vi "String to I8.vi"(8 "Error In":errorcluster, 11 "String":string) -> (0 "Error Out":errorcluster, 2 "I8":i8, 3 "rest of String":string)   [LabVIEW 2011, in "Tinkerforge.lvlib" / "Device.lvclass"]
doc: "This VI converts a binary little-endian I8 string into a numeric I8."
uses:
  Device.lvclass
  IP Connection/IP Connection.lvclass
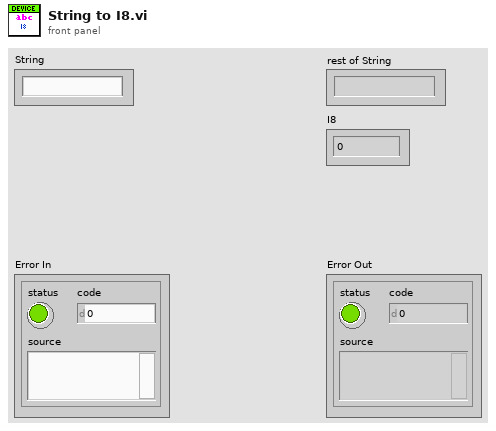
[diagram p1: front panel]
types:
  T1 = enum16{"big-endian, network order", "native, host order", "little-endian"}
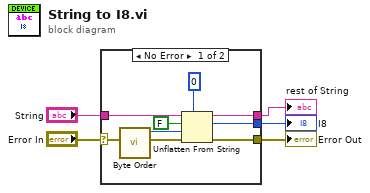
[diagram p0: block diagram]
diagram:
  n1 = case shown="No Error" "Error In" {
    selector: "Error In" -> [w12 w15]
    tunnel: "String" -> [w9 w14]
    tunnel: [w8 w15] -> w3
    tunnel: [w7 _] -> w2
    tunnel: [w6 w14] -> w1
    frame No Error {
      n2 = call "Byte Order.vi"() -> ("byte order (2:little-endian)"=w11:T1)  [unwired: 11 in]
      n3 = Unflatten From String(type=i8 0, binary string=w9, data includes array or string size? (T)=FALSE, byte order (0:big-endian, network order)=w11, error in (no error)=w12) -> (rest of the binary string=w6:string, value=w7:i8, error out=w8:errorcluster)
    }
    frame Error {
    }
  }
  "Error Out" <- w3
  "I8" <- w2
  "rest of String" <- w1
